vi "XXPathPlanner_RotationTarget_ForSegmentIndex.vi"(9 "SegmentIndex":i32, 11 "RotationTarget":T1={"position"=0.0, "rotation"={"VALUE"=0.0, "COS"=1.0, "SIN"=0.0}, "Exists"=FALSE} {"rotation"."SIN" format="%13.4f"; "rotation"."COS" format="%13.4f"; "rotation"."VALUE" format="%13.4f"}) -> (3 "new RotationTarget":T1={"position"=0.0, "rotation"={"VALUE"=0.0, "COS"=1.0, "SIN"=0.0}, "Exists"=FALSE} {"rotation"."SIN" format="%13.4f"; "rotation"."COS" format="%13.4f"; "rotation"."VALUE" format="%13.4f"})   [LabVIEW 2019]
doc: "Transform the position of this target for a given segment number.\n \nFor example, a target with position 1.5 for the segment 1 will have the position 0.5\n \nInputs: \n - RotationTarget - cluster - defined rotation target data structure\n - segmentIndex- integer - The segment index to transform position for\n\nOutputs:\n - NewRotationTarget - cluster - The transformed target"
uses:
  TypeDef/PathPlannerRotationTarget.ctl
  <vilib>/Rock Robotics/WPI/ThirdParty/JAS_Junk/TrajLib/TypeDef/ROTATION2D.ctl
  PathPlanner24.lvlib
  <vilib>/Rock Robotics/WPI/ThirdParty/JAS_Junk/TrajLib/Trajectory_Library.lvlib
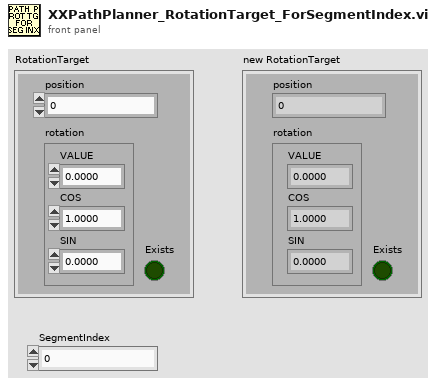
[diagram p1: front panel]
types:
  T1 = typedef "PathPlanner24.lvlib/PathPlannerRotationTarget.ctl" = cluster{"position":dbl, "rotation":T2, "Exists":bool}
  T2 = typedef "Trajectory_Library.lvlib/ROTATION2D.ctl" = cluster{"VALUE":dbl, "COS":dbl, "SIN":dbl}
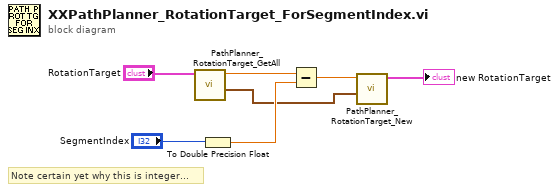
[diagram p0: block diagram]
diagram:
  # "Note certain yet why this is integer..."
  n1 = call "PathPlanner_RotationTarget_GetAll.vi"("RotationTarget"="RotationTarget") -> ("rotation"=w3:T2, "position"=w5:dbl)  [unwired: 8 in, 1 out]
  n2 = To Double Precision Float(number="SegmentIndex") -> (double precision float=w4:dbl)
  n3 = Subtract(x=w5, y=w4) -> (x-y=w2:dbl)
  n4 = call "PathPlanner_RotationTarget_New.vi"("rotation"=w3, "position"=w2) -> ("RotationTarget"=→"new RotationTarget":T1)  [unwired: 9 in]
